vi "Pre Loop Init.vi"(8 "Error In":errorcluster, 11 "This VI":refnum<vi>) -> (0 "Error Out":errorcluster, 3 "Event Registration Refnum":refnum<event-registration>)   [LabVIEW 2015, in "Config DB.lvlib"]
doc: "VI used to load initial parameters for this module."
uses:
  Config DB.lvlib
  Private Controls/Module Data Cluster.ctl
  Private Controls/Module Action.ctl
  User Events/Controls/User Events States.ctl
  Private Controls/Queue FGV Action.ctl
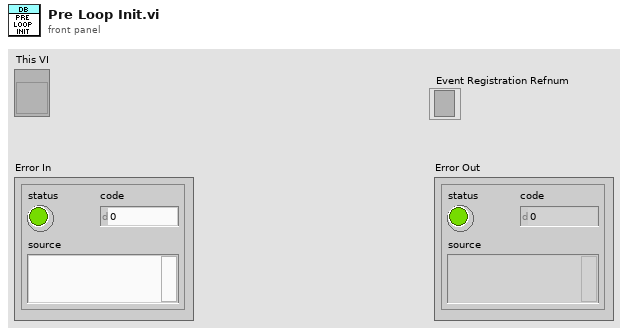
[diagram p1: front panel]
types:
  T1 = typedef "Config DB.lvlib/Queue FGV Action.ctl" = enum16{"Set", "Get", "Release"}
  T2 = typedef "User Events States.ctl" = enum16{"Get", "Create", "Destroy"}
  T3 = typedef "Config DB.lvlib/Module Data Cluster.ctl" = cluster{"Data":variant, "Action":T4}
  T4 = typedef "Config DB.lvlib/Module Action.ctl" = enum16{"Init", "Close", "Error"}
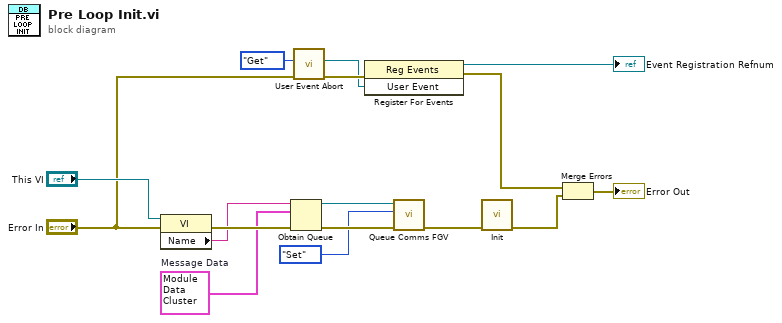
[diagram p0: block diagram]
diagram:
  w13 = T3 {"Data"=variant, "Action"=enum."Init"}  # Message Data
  n1 = property class="VI"(reference="This VI", error in="Error In") -> (error out=w15:errorcluster, "Name"=w14:string)  [unwired: 1 out]
  n2 = Obtain Queue(name (unnamed)=w14, element data type=w13, error in (no error)=w15) -> (queue out=w6:refnum<queue>, error out=w7:errorcluster)  [unwired: 2 in, 1 out]
  n3 = call "User Event Abort.vi"("Error In"="Error In", "User Event States"=User_Events_States."Get") -> ("Error Out"=w10:errorcluster, "User Event"=w9:refnum<user-event>)  [unwired: 8 in]
  n4 = register-events(error in=w10, w9) -> (reference out=→"Event Registration Refnum":refnum<event-registration>, error out=w3:errorcluster)  [unwired: 1 in]
  n5 = call "Queue Comms FGV.vi"("Error In"=w7, "Queue Option"=Queue_FGV_Action."Set", "Queue In"=w6) -> ("Error Out"=w4:errorcluster)  [unwired: 7 in, 1 out]
  n6 = call "Init.vi"("Error In"=w4) -> ("Error Out"=w2:errorcluster)  [unwired: 10 in]
  n7 = Merge Errors(w3, w2) -> (→"Error Out":errorcluster)
